vi "Run Protocol.vi"(8 "error in (no error)":errorcluster, 10 "Protocol In":T4={"Camera Settings"={"Exposure Time (ms)"=100.0, "Binning"=enum."2x2", "Scan Mode"=0, "Frames to Acquire"=1000.0, "Pixel Correction"=FALSE, "Frames to Skip"=0, "File Path"=path "", "Duty cycle"=0.0, "ALEX"=FALSE, "Shutter Enable"=[], "fluidics trigger, ms (0=disabled)"=0.0, "Bit Depth"=0, "Image Width (px)"=0, "Image Height (px)"=0, "Horizontal Offset (px)"=0, "Vertical Offset (px)"=0}, "Auto-Advance"=TRUE, "Auto Focus"=TRUE, "Injection Countdown"=TRUE, "Fields"=1, "Lanes"=1, "Acquisition type"=enum."Movie series", "Particle Count Threshold"=0} {"Camera Settings"."Exposure Time (ms)" min=1.0 max=10000.0 step=1.0}, 11 "AutomationContext in":refnum<class "AutomationContext.lvclass">) -> (0 "error out":errorcluster, 3 "AutomationContext out":refnum<class "AutomationContext.lvclass">)   [LabVIEW 2023, in "Automation.lvlib" / "AutomationContext.lvclass"]
uses:
  AutomationContext.lvclass
  Resources/Type Defs/Movie Series.ctl
  Resources/Type Defs/Camera Settings.ctl
  Resources/Type Defs/Movie auto-numbering.ctl
  Parallel Block.ctl
  Automation Intent.ctl
  Intent Action.ctl
  AutomationContext.lvclass/AutomationContext.ctl
panel:
  out "Run Plan":T1[](array[typedef])
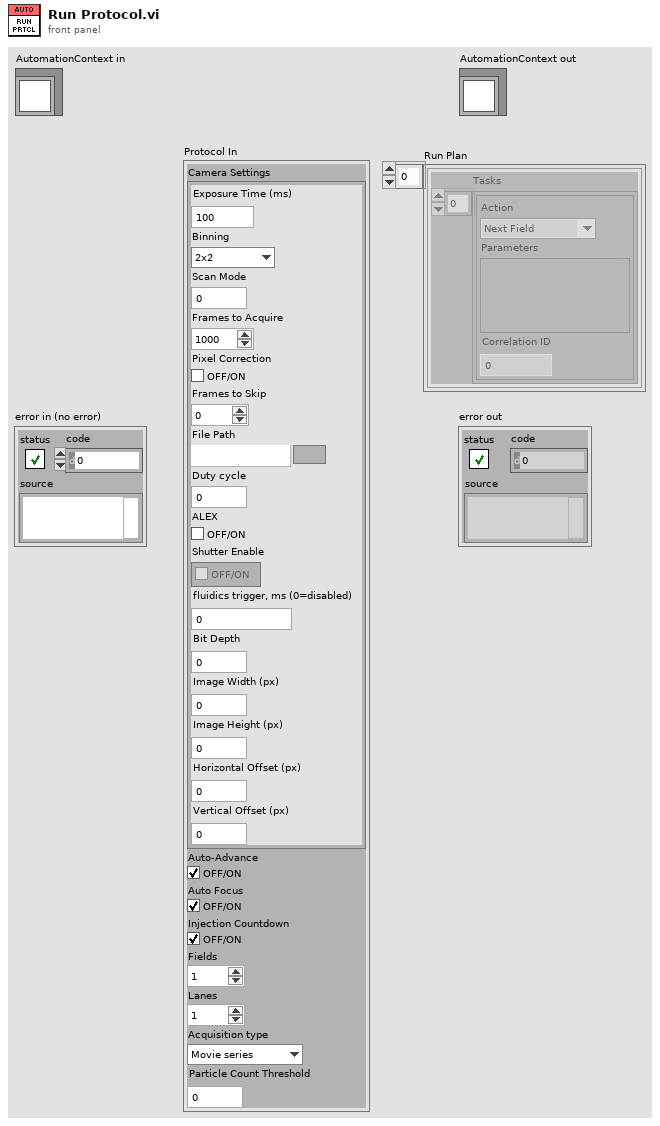
[diagram p1: front panel]
types:
  T1 = typedef "Automation.lvlib/AutomationContext.lvclass/Parallel Block.ctl" = cluster{"Tasks":T2[]}
  T2 = typedef "Automation.lvlib/AutomationContext.lvclass/Automation Intent.ctl" = cluster{"Action":T3, "Parameters":variant, "Correlation ID":u32}
  T3 = typedef "Automation.lvlib/AutomationContext.lvclass/Intent Action.ctl" = enum16{"Next Field", "Next Lane", "Set Power", "Reset Power", "Autofocus", "Start Streaming", "Delay", "Finish Run", "Open Shutter", "Close Shutter"}
  T4 = typedef "Movie Series.ctl" = cluster{"Camera Settings":T5, "Auto-Advance":bool, "Auto Focus":bool, "Injection Countdown":bool, "Fields":i32, "Lanes":i32, "Acquisition type":T6, "Particle Count Threshold":i32}
  T5 = typedef "Camera Settings.ctl" = cluster{"Exposure Time (ms)":dbl, "Binning":enum16{"1x1", "2x2", "4x4"}, "Scan Mode":i32, "Frames to Acquire":dbl, "Pixel Correction":bool, "Frames to Skip":u32, "File Path":path, "Duty cycle":dbl, "ALEX":bool, "Shutter Enable":bool[], "fluidics trigger, ms (0=disabled)":dbl, "Bit Depth":u16, "Image Width (px)":u16, "Image Height (px)":u16, "Horizontal Offset (px)":u16, "Vertical Offset (px)":u16}
  T6 = typedef "Movie auto-numbering.ctl" = enum16{"Single movie", "Movie series", "Multi-lane series"}
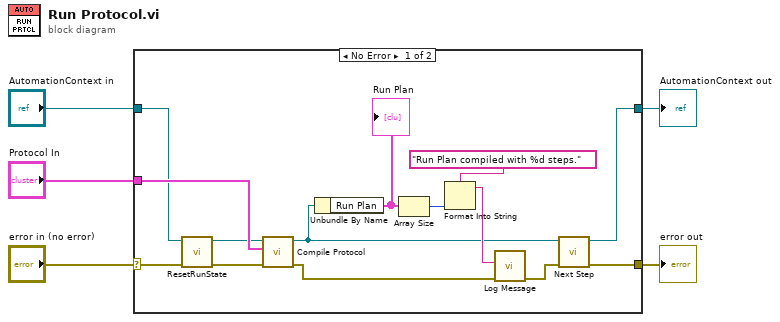
[diagram p0: block diagram]
diagram:
  n1 = case shown="No Error" "error in (no error)" {
    selector: "error in (no error)" -> [w10 w21]
    tunnel: [w19 w21] -> w4
    tunnel: [w18 w20] -> w2
    tunnel: "AutomationContext in" -> [w7 w20]
    tunnel: "Protocol In" -> [w17 _]
    frame No Error {
      n2 = call "ResetRunState.vi"("error in (no error)"=w10, "AutomationContext in"=w7) -> ("error out"=w9:errorcluster, "AutomationContext out"=w8:refnum<class "AutomationContext.lvclass">)  [unwired: 8 in]
      n3 = call "Compile Protocol.vi"("error in (no error)"=w9, "Protocol In"=w17, "AutomationContext in"=w8) -> ("error out"=w16:errorcluster, "AutomationContext out"=w6:refnum<class "AutomationContext.lvclass">)  [unwired: 7 in]
      n4 = Unbundle By Name(w6) -> ("Run Plan"=w13:T1[])
      "Run Plan" <- w13
      n5 = Array Size(array=w13) -> (size(s)=w12:i32)
      n6 = Format Into String(format string="Run Plan compiled with %d steps." ("input"), w12) -> (resulting string=w11:string)  [unwired: 2 in, 1 out]
      n7 = call "Log Message.vi"("error constant"=w16, "input"=w11) -> ("error constant 2"=w15:errorcluster)  [unwired: 8 in, 1 out]
      n8 = call "Next Step.vi"("error in (no error)"=w15, "AutomationContext in"=w6) -> ("error out"=w19:errorcluster, "AutomationContext out"=w18:refnum<class "AutomationContext.lvclass">)  [unwired: 8 in]
    }
    frame Error {
    }
  }
  "error out" <- w4
  "AutomationContext out" <- w2
